vi "util-ini-key.vi"(10 "key":T1=enum."INI.ENV", 11 "section":T2) -> (2 "key":string, 3 "section":string)   [LabVIEW 2024]
uses:
  controls/ini-section.ctl
  controls/ini-key.ctl
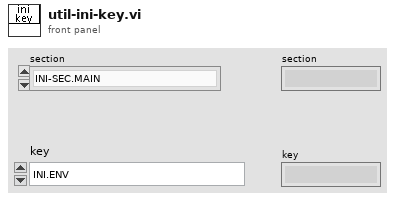
[diagram p1: front panel]
types:
  T1 = typedef "ini-key.ctl" = enum16{"INI.PROJECT_NAME", "INI.ENV", "INI.ENG.SERIAL", "INI.ENG.INTERVAL_MS", "INI.LOCAL.LONGITUDE", "INI.LOCAL.LATITUDE", "INI.LOCAL.TIMEZONE"}
  T2 = typedef "ini-section.ctl" = enum16{"INI-SEC.MAIN"}
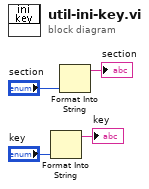
[diagram p0: block diagram]
diagram:
  n1 = Format Into String("key") -> (resulting string=→"key":string)  [unwired: 3 in, 1 out]
  n2 = Format Into String("section") -> (resulting string=→"section":string)  [unwired: 3 in, 1 out]
